vi "Test UNSUBSCRIBE packet.vi"(8 "error in":errorcluster) -> (0 "error out":errorcluster)   [LabVIEW 2013]
uses:
  source/Control Packets/UNSUBSCRIBE/UNSUBSCRIBE.lvclass
  source/Control Packets/ControlPacket/ControlPacket.lvclass/ControlPacket.ctl
  source/Control Packets/ControlPacket/ControlPacket.lvclass
  <vilib>/addons/_JKI Toolkits/Caraya/classes/Test/Test.lvclass
  <vilib>/addons/_JKI Toolkits/Caraya/classes/Assert/Assert.lvclass
panel:
  out "Payload":u8[](array[numeric])
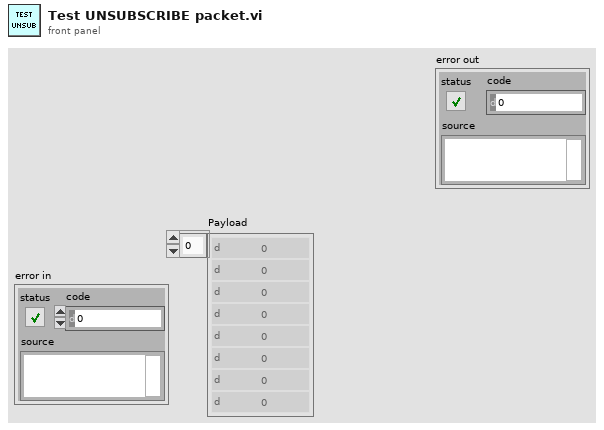
[diagram p1: front panel]
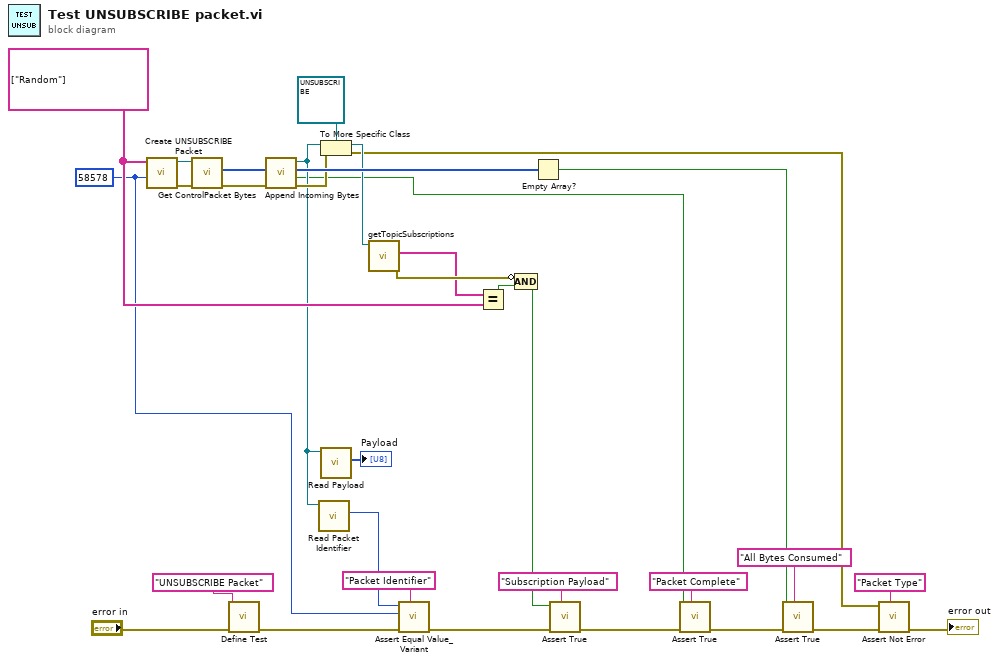
[diagram p0: block diagram]
diagram:
  w26 = string[] ["Random"] ("Topic Subscriptions")
  w5 = u16 58578 ("Packet ID")
  n1 = call "Create UNSUBSCRIBE Packet.vi"("Packet ID (0: generate new)"=w5, "Topic Subscriptions"=w26) -> ("error out"=w28:errorcluster, "UNSUBSCRIBE out"=w27:refnum<class "UNSUBSCRIBE.lvclass">)  [unwired: 8 in]
  n2 = call "Get ControlPacket Bytes.vi"("error in (no error)"=w28, "ControlPacket"=w27) -> ("error out"=w31:errorcluster, "Bytes Stream"=w33:u8[])  [unwired: 6 in, 2 out]
  n3 = call <vilib>:"Define Test.vi"("error in (no error)"="error in", "Label (VI Title)"="UNSUBSCRIBE Packet") -> ("error out"=w14:errorcluster)  [unwired: 9 in]
  n4 = call "Append Incoming Bytes.vi"("error in (no error)"=w31, "Incoming Packets"=w33) -> ("error out"=w30:errorcluster, "Complete Packet"=w7:bool, "Remaining Packets"=w32:u8[], "ControlPacket"=w22:refnum<class "ControlPacket.lvclass">)  [unwired: 6 in]
  n5 = call "Read Packet Identifier.vi"("ControlPacket in"=w22) -> ("Packet Identifier"=w6:u16)  [unwired: 9 in, 1 out]
  n6 = To More Specific Class(target class=refnum<class "UNSUBSCRIBE.lvclass"> refnum ("MQTT_Control_Packets.lvlib:UNSUBSCRIBE.lvclass"), reference=w22, error in=w30) -> (specific class reference=w25:refnum<class "UNSUBSCRIBE.lvclass">, error out=w10:errorcluster)
  n7 = call "Read Payload.vi"("ControlPacket in"=w22) -> ("Payload"=→"Payload":u8[])  [unwired: 9 in, 1 out]
  n8 = call "getTopicSubscriptions.vi"("UNSUBSCRIBE in"=w25) -> ("error out"=w24:errorcluster, "Topic Subscriptions"=w23:string[])  [unwired: 8 in, 1 out]
  n9 = call <vilib>:"Assert Equal Value_Variant.vi"("Label"="Packet Identifier" ("Label (VI Title)"), "error in (no error)"=w14, "Y"=w5, "X"=w6) -> ("error out"=w3:errorcluster)  [unwired: 7 in]
  n10 = Equal?(x=w23, y=w26) -> (x = y?=w29:bool)
  n11 = Compound Arithmetic op=AND(invert w24, w29) -> (w1:bool)
  n12 = Empty Array?(array=w32) -> (empty?=w8:bool)
  n13 = call <vilib>:"Assert True.vi"("Label"="Subscription Payload" ("Label (VI Title)"), "error in (no error)"=w3, "True?"=w1) -> ("error out"=w2:errorcluster)  [unwired: 8 in]
  n14 = call <vilib>:"Assert True.vi"("Label"="Packet Complete" ("Label (VI Title)"), "error in (no error)"=w2, "True?"=w7) -> ("error out"=w15:errorcluster)  [unwired: 8 in]
  n15 = call <vilib>:"Assert True.vi"("Label"="All Bytes Consumed" ("Label (VI Title)"), "error in (no error)"=w15, "True?"=w8) -> ("error out"=w12:errorcluster)  [unwired: 8 in]
  n16 = call <vilib>:"Assert Not Error.vi"("Label"="Packet Type" ("Label (VI Title)"), "error in (no error)"=w12, "Not Error?"=w10) -> ("error out"=→"error out":errorcluster)  [unwired: 8 in]
